vi "VisionAlign.vi"(11 "HoldingCargo":bool) -> (1 "Z":dbl, 2 "Y":dbl, 3 "X":dbl)   [LabVIEW 2018]
uses:
  <vilib>/Rock Robotics/Network Tables/NT Read Numeric Array.vi
  Globals.vi
panel:
  in  "Turning scale factor":dbl=0.06
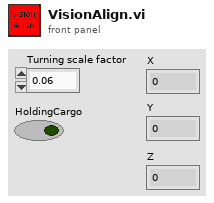
[diagram p1: front panel]
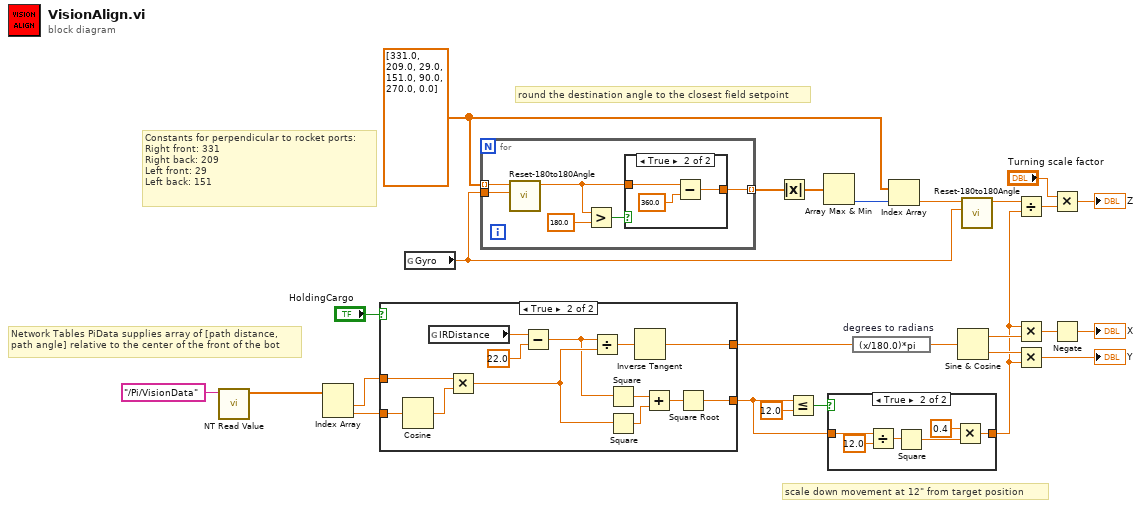
[diagram p0: block diagram]
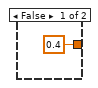
[diagram p2: hidden frame]
diagram:
  w18 = dbl[] [331.0, 209.0, 29.0, 151.0, 90.0, 270.0, 0.0]
  # "scale down movement at 12\" from target position"
  # "round the destination angle to the closest field setpoint"
  # "Network Tables PiData supplies array of [path distance,\npath angle] relative to the center of the front of the bot"
  # "Constants for perpendicular to rocket ports:\nRight front: 331\nRight back: 209\nLeft front: 29\nLeft back: 151"
  n1 = call-poly <vilib>:"NT Read Value.vi"("Name"="/Pi/VisionData" ("Client Name")) -> ("Numeric Array"=w25:dbl[])  [unwired: 9 in, 1 out]
  n2 = Index Array(array=w25) -> (element #1=w10:dbl, element #2=w8:dbl)  [unwired: 2 in]
  n3 = case shown="True" "HoldingCargo" {
    tunnel: [w28 w31] -> w4
    tunnel: w10 -> [w28 w39]
    tunnel: [w27 w35] -> w9
    tunnel: w8 -> [w27 w41]
    frame False {
    }
    frame True {
      n4 = Cosine(x=w41) -> (cos(x)=w40:dbl)
      n5 = global read "Globals.vi" "IRDistance"() -> (w38:dbl)
      n6 = Multiply(x=w39, y=w40) -> (x*y=w30:dbl)
      n7 = Subtract(x=w38, y=22.0) -> (x-y=w29:dbl)
      n8 = Divide(x=w29, y=w30) -> (x/y=w36:dbl)
      n9 = Square(x=w29) -> (x^2=w34:dbl)
      n10 = Square(x=w30) -> (x^2=w33:dbl)
      n11 = Inverse Tangent(1:w36) -> (0:w35:dbl)
      n12 = Add(x=w34, y=w33) -> (x+y=w32:dbl)
      n13 = Square Root(x=w32) -> (sqrt(x)=w31:dbl)
    }
  }
  n14 = global read "Globals.vi" "Gyro"() -> (w1:dbl)
  n15 = for {
    tunnel: w18 -> [w47] mode=indexing
    tunnel: w1 -> [w46]
    tunnel: [w45] -> w19 mode=indexing
    n16 = call "Reset-180to180Angle.vi"("Offset"=w46, "AngleInput"=w47) -> ("AngleOutput"=w44:dbl)  [unwired: 9 in]
    n17 = Greater?(x=w44, y=180.0) -> (0:w42:bool)
    n18 = case shown="True" w42 {
      tunnel: w44 -> [w48 w50]
      tunnel: [w48 w49] -> w45
      frame False {
      }
      frame True {
        n19 = Subtract(x=w50, y=360.0) -> (x-y=w49:dbl)
      }
    }
  }
  n20 = Absolute Value(x=w19) -> (abs(x)=w23:dbl[])
  n21 = Less Or Equal?(x=w4, y=12.0) -> (x <= y?=w6:bool)
  n22 = Array Max & Min(array=w23) -> (min index (indices)=w22:i32)  [unwired: 3 out]
  n23 = case shown="True" w6 {
    tunnel: w4 -> [_ w58]
    tunnel: [0.4 w54] -> w3
    frame False {
    }
    frame True {
      n24 = Divide(x=w58, y=12.0) -> (x/y=w53:dbl)
      n25 = Square(x=w53) -> (x^2=w56:dbl)
      n26 = Multiply(x=0.4, y=w56) -> (x*y=w54:dbl)
    }
  }
  n27 = expression code="(x/180.0)*pi" "degrees to radians"(w9) -> (w24:dbl)
  n28 = Index Array(array=w18, index=w22) -> (element=w17:dbl)
  n29 = Sine & Cosine(0:w24) -> (1:w21:dbl, 2:w20:dbl)
  n30 = call "Reset-180to180Angle.vi"("Offset"=w1, "AngleInput"=w17) -> ("AngleOutput"=w5:dbl)  [unwired: 9 in]
  n31 = Divide(x=w5, y=w3) -> (x/y=w16:dbl)
  n32 = Multiply(x=w3, y=w21) -> (x*y=w12:dbl)
  n33 = Multiply(x=w20, y=w3) -> (x*y=→"Y":dbl)
  n34 = Multiply(x="Turning scale factor", y=w16) -> (x*y=→"Z":dbl)
  n35 = Negate(x=w12) -> (-x=→"X":dbl)
